vi "Transform.vi"(7 "Type X":T2(ring), 8 "error in (no error)":errorcluster caption="entrée d'erreur (pas d'erreur)", 9 "y":string[][](array[string]), 10 "X":string[][](array[string]), 11 "SimpleImputer.lvclass":refnum<class "SimpleImputer.lvclass">) -> (0 "error out":errorcluster caption="sortie d'erreur", 2 "Data":T1, 3 "SimpleImputer.lvclass":refnum<class "SimpleImputer.lvclass">)   [LabVIEW 2020, in "SimpleImputer.lvclass"]
doc: "Impute all missing values in X.\n\nReturns : \n\n- X : {array-like, sparse matrix}, shape (n_samples, n_features)\nThe input data to complete."
uses:
  SimpleImputer.lvclass
  SimpleImputer.lvclass/SimpleImputer.ctl
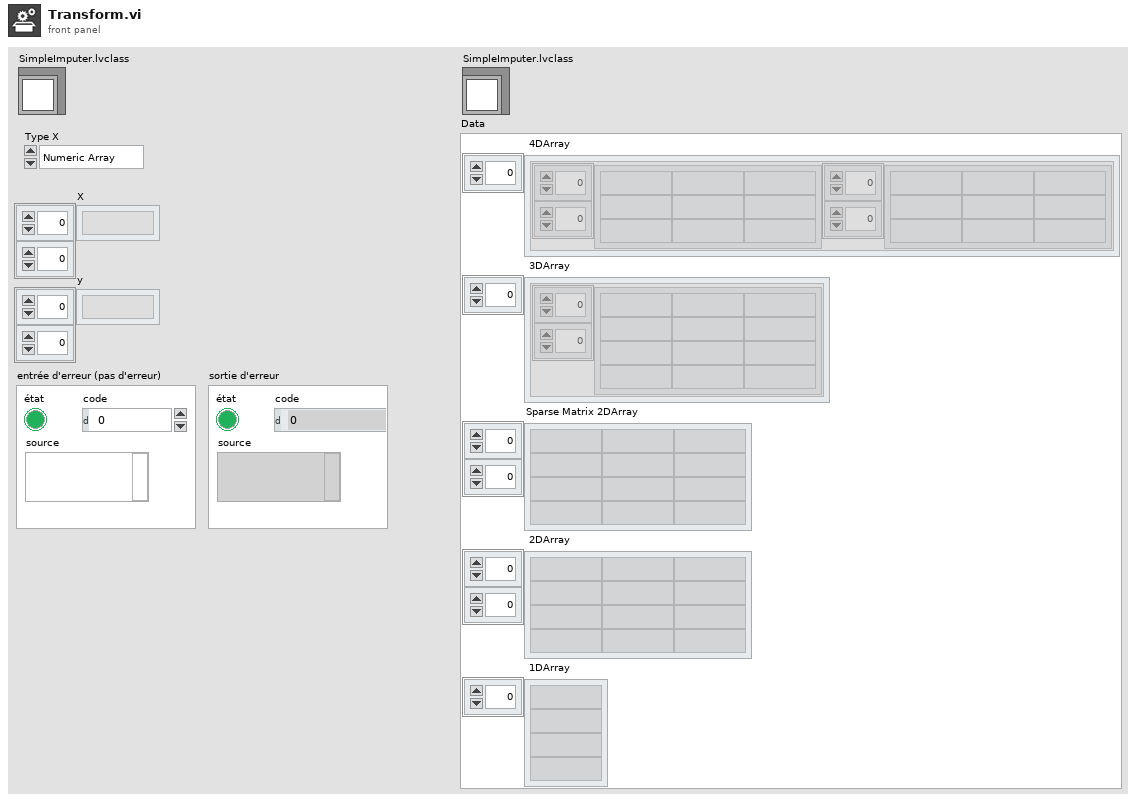
[diagram p1: front panel]
types:
  T1 = cluster{" 4DArray":cluster{"1":string[][], "2":string[][]}[], " 3DArray":cluster{"Tableau":string[][]}[], "Sparse Matrix 2DArray":string[][], " 2DArray":string[][], " 1DArray":string[]}
  T2 = enum16{"Numeric Array", "String Array", "Sparse"}
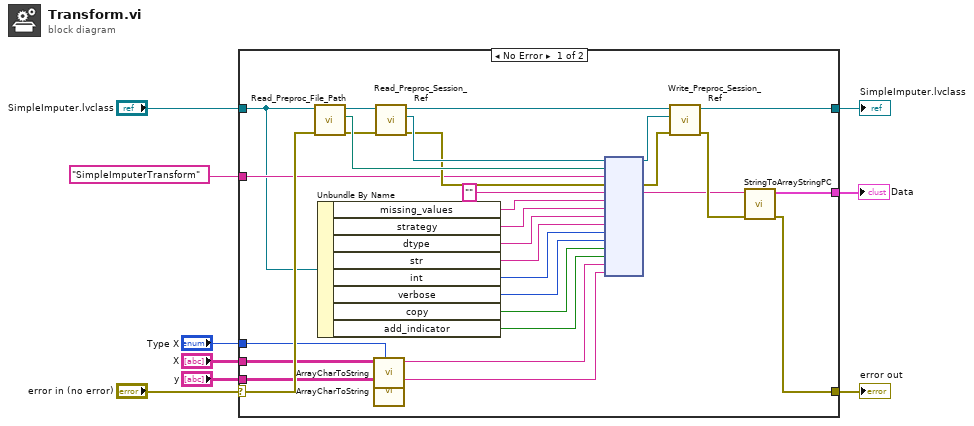
[diagram p0: block diagram]
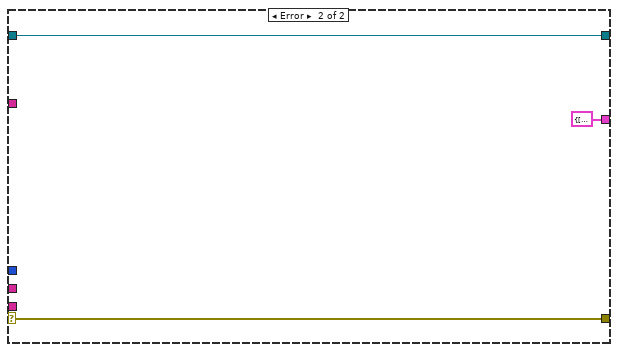
[diagram p2: hidden frame]
diagram:
  n1 = case shown="No Error" "error in (no error)" {
    selector: "error in (no error)" -> [w30 w42]
    tunnel: [w16 w42] -> w8
    tunnel: [w29 w41] -> w6
    tunnel: "SimpleImputer.lvclass" -> [w27 w41]
    tunnel: "SimpleImputerTransform" ("Fonction") -> [w28 _]
    tunnel: "X" -> [w14 _]
    tunnel: "y" -> [w11 _]
    tunnel: [w15 T1 {" 4DArray"=[], " 3DArray"=[], "Sparse Matrix 2DArray"=[], " 2DArray"=[], " 1DArray"=[]} ("Data")] -> w2
    tunnel: "Type X" -> [w13 _]
    frame No Error {
      n2 = call-dynamic "Read_Preproc_File_Path.vi"("error in (no error)"=w30, "Python in"=w27) -> ("error out"=w34:errorcluster, "File_Path"=w37:path, "Python out"=w39:refnum<class "SimpleImputer.lvclass">)  [unwired: 7 in]
      n3 = Unbundle By Name(w27) -> ("missing_values"=w26:string, "strategy"=w25:string, "dtype"=w24:string, "str"=w23:string, "int"=w22:i32, "verbose"=w21:i32, "copy"=w20:bool, "add_indicator"=w19:bool)
      n4 = call "ArrayCharToString.vi"("Type"=w13, "TAB"=w14) -> ("Instruction"=w12:string)  [unwired: 9 in]
      n5 = call "ArrayCharToString.vi"("TAB"=w11) -> ("Instruction"=w10:string)  [unwired: 10 in]
      n6 = call-dynamic "Read_Preproc_Session_Ref.vi"("error in (no error)"=w34, "Python in"=w39) -> ("error out"=w35:errorcluster, "Session_ref"=w36:refnum<k35>, "Python out"=w38:refnum<class "SimpleImputer.lvclass">)  [unwired: 7 in]
      n7 = node(w36, w37, w28, w35, "", w26, w25, w24, w23, w22, w21, w20, w19, w12, w10) -> (w31:refnum<k35>, w33:errorcluster, w17:string)  [unwired: 10 in, 2 out]
      n8 = call-dynamic "Write_Preproc_Session_Ref.vi"("error in (no error)"=w33, "Session_ref"=w31, "Python in"=w38) -> ("error out"=w18:errorcluster, "Python out"=w29:refnum<class "SimpleImputer.lvclass">)  [unwired: 7 in]
      n9 = call "StringToArrayStringPC.vi"("sortie d'erreur"=w18, "Return value"=w17) -> ("sortie d'erreur"=w16:errorcluster, "Data"=w15:T1)  [unwired: 8 in]
    }
    frame Error {
    }
  }
  "error out" <- w8
  "SimpleImputer.lvclass" <- w6
  "Data" <- w2
